vi "new Door.vi"(8 "error in (no error)":errorcluster, 9 "r2":refnum<data-value>, 10 "r1":refnum<data-value>) -> (0 "error out":errorcluster, 3 "Door* out":refnum<data-value>)   [LabVIEW 2016, in "Door.lvclass"]
uses:
  Door.lvclass
  Room/Room.lvclass
  Door.lvclass/Door.ctl
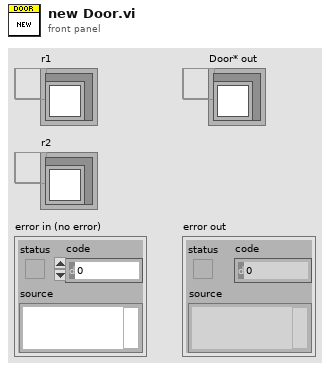
[diagram p1: front panel]
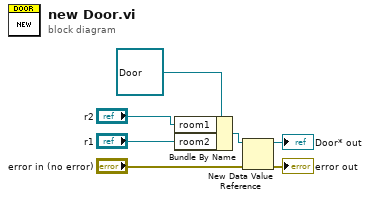
[diagram p0: block diagram]
diagram:
  n1 = Bundle By Name(cluster=refnum<class "Door.lvclass"> refnum ("Door in"), "room1"="r2", "room2"="r1") -> (w4:refnum<class "Door.lvclass">)
  n2 = New Data Value Reference(data value=w4, error in="error in (no error)") -> (data value reference=→"Door* out":refnum<data-value>, error out=→"error out":errorcluster)
